vi "Initialize.vi"(8 "error in (no error)":errorcluster, 11 "View Template in":refnum<class "[V] Sys Cfg Main.lvclass">) -> (0 "error out":errorcluster, 3 "View Template out":refnum<class "[V] Sys Cfg Main.lvclass">)   [LabVIEW 2020, in "[V] Sys Cfg Main.lvlib" / "[V] Sys Cfg Main.lvclass"]
uses:
  [V] Sys Cfg Main.lvclass
  [V] Sys Cfg Main.lvclass/[V] Sys Cfg Main.ctl
  [V] Sys Cfg Base/[V] Sys Cfg Base/[V] Sys Cfg Base.lvclass
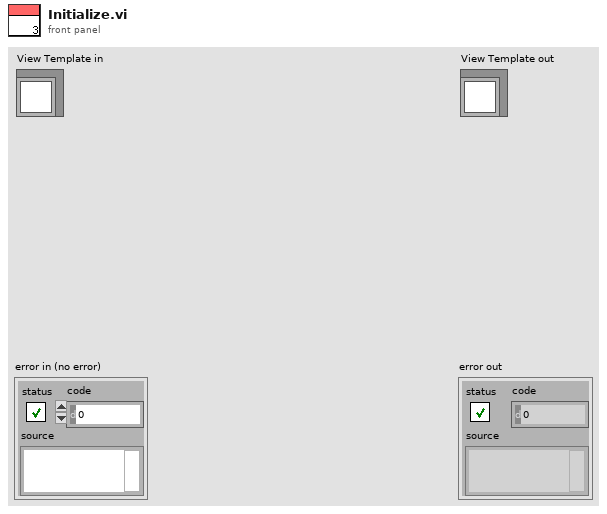
[diagram p1: front panel]
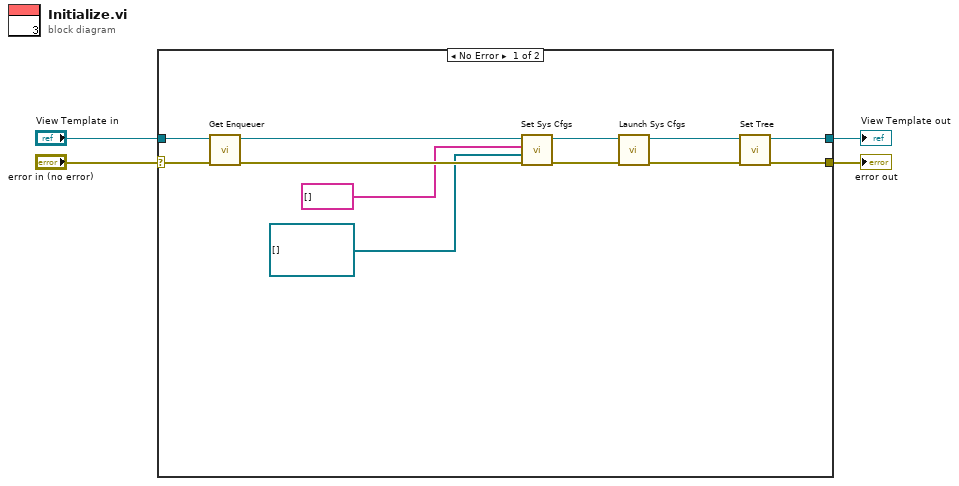
[diagram p0: block diagram]
diagram:
  n1 = case shown="No Error" "error in (no error)" {
    selector: "error in (no error)" -> [w15 w18]
    tunnel: [w13 w18] -> w3
    tunnel: [w11 w17] -> w1
    tunnel: "View Template in" -> [w16 w17]
    frame No Error {
      n2 = call "Get Enqueuer.vi"("error in (no error)"=w15, "View Template in"=w16) -> ("error out"=w7:errorcluster, "View Template out"=w10:refnum<class "[V] Sys Cfg Main.lvclass">)  [unwired: 8 in]
      n3 = call "Set Sys Cfgs.vi"("error in (no error)"=w7, "sys cfgs"=refnum<class "[V] Sys Cfg Base.lvclass">[] [], "names"=string[] [], "[V] Sys Cfg Main in"=w10) -> ("error out"=w8:errorcluster, "[V] Sys Cfg Main out"=w9:refnum<class "[V] Sys Cfg Main.lvclass">)  [unwired: 6 in]
      n4 = call "Launch Sys Cfgs.vi"("error in (no error)"=w8, "[V] Sys Cfg Main in"=w9) -> ("error out"=w14:errorcluster, "[V] Sys Cfg Main out"=w12:refnum<class "[V] Sys Cfg Main.lvclass">)  [unwired: 8 in]
      n5 = call "Set Tree.vi"("error in (no error)"=w14, "[V] Sys Cfg Main in"=w12) -> ("error out"=w13:errorcluster, "[V] Sys Cfg Main out"=w11:refnum<class "[V] Sys Cfg Main.lvclass">)  [unwired: 8 in]
    }
    frame Error {
    }
  }
  "error out" <- w3
  "View Template out" <- w1
